vi "Execute.vi"(8 "error in (no error)":errorcluster, 9 "System in":refnum<class "System.lvclass">, 10 "Command in":refnum<class "Command.lvclass">, 11 "BL-Retracting-State in":refnum<class "BL-Retracting-State.lvclass">) -> (0 "error out":errorcluster, 2 "Next State":refnum<class "State.lvclass">, 3 "BL-Retracting-State out":refnum<class "BL-Retracting-State.lvclass">)   [LabVIEW 2013, in "BL-Retracting-State.lvclass"]
uses:
  BL-Retracting-State.lvclass
  Commands/Command/Command.lvclass
  Systems/System/System.lvclass
  State/State.lvclass
  Systems/Blocker/Blocker.lvclass
  Robot Global Data.vi
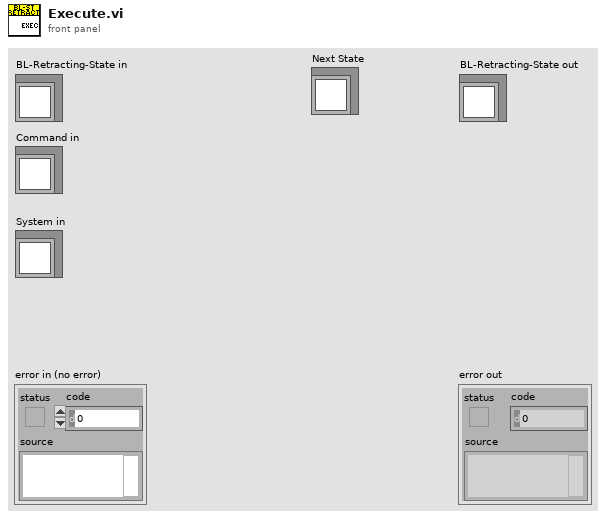
[diagram p1: front panel]
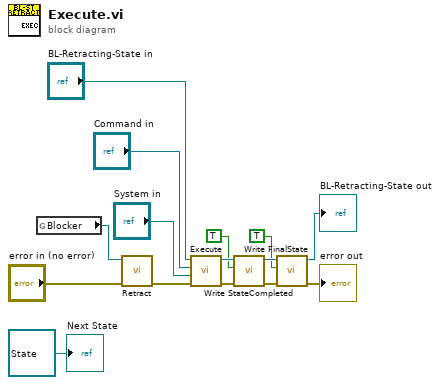
[diagram p0: block diagram]
diagram:
  n1 = global read "Robot Global Data.vi" "Blocker"() -> (w11:refnum<class "Blocker.lvclass">)
  n2 = call-dynamic "Retract.vi"("error in (no error)"="error in (no error)", "Blocker in"=w11) -> ("error out"=w9:errorcluster)  [unwired: 8 in, 1 out]
  n3 = call-parent "Execute.vi"("error in (no error)"=w9, "System in"="System in", "Command in"="Command in", "State in"="BL-Retracting-State in") -> ("error out"=w3:errorcluster, "State out"=w8:refnum<class "BL-Retracting-State.lvclass">)  [unwired: 5 in, 1 out]
  n4 = call-dynamic "Write StateCompleted.vi"("error in (no error)"=w3, "StateCompleted"=TRUE, "State in"=w8) -> ("error out"=w2:errorcluster, "State out"=w7:refnum<class "BL-Retracting-State.lvclass">)  [unwired: 7 in]
  n5 = call-dynamic "Write FinalState.vi"("error in (no error)"=w2, "FinalState"=TRUE, "State in"=w7) -> ("error out"=→"error out":errorcluster, "State out"=→"BL-Retracting-State out":refnum<class "BL-Retracting-State.lvclass">)  [unwired: 7 in]
  "Next State" <- refnum<class "State.lvclass"> refnum ("State.lvclass")
